vi "IP Reporter PythonCode Folder.vi"() -> ()   [LabVIEW 2017]
doc: "Opens the folder holding the IP Reporter Python sources in the default file browser."
uses:
  <vilib>/Platform/browser.llb/Open URL in Default Browser (path).vi
panel:
  out "PythonCode":path
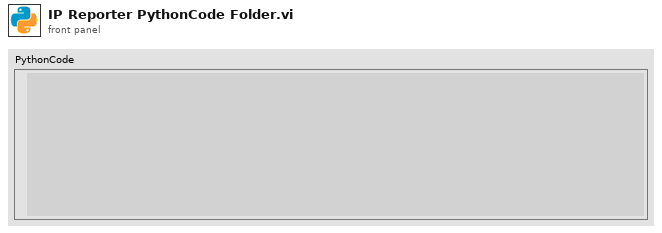
[diagram p1: front panel]
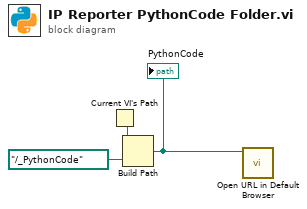
[diagram p0: block diagram]
diagram:
  n1 = Current VI's Path() -> (path=w3:path)
  n2 = Build Path(base path=w3, name or relative path=path "../_PythonCode") -> (appended path=w1:path)
  "PythonCode" <- w1
  n3 = call-poly <vilib>:"Open URL in Default Browser.vi"("path"=w1) -> ()  [unwired: 5 in, 2 out]
